vi "Create.vi"(8 "ErrorArray":errorcluster[](array[cluster]), 10 "name or relative path":string="PARTF\\PARTF.ini") -> (0 "ErrorArray":errorcluster[](array[cluster]), 3 "Ref out":refnum<class "Config.lvclass">)   [LabVIEW 2017, in "Framework.lvlib" / "Config.lvclass"]
uses:
  Config.lvclass
  <vilib>/Utility/sysdir.llb/System Directory Type.ctl
  Typedefs/RootDir.ctl
  Typedefs/Logging.ctl
  Typedefs/eLogLvl.ctl
  Config.lvclass/Config.ctl
  Accessors/Write ConfigFilePath.vi
  Accessors/Write Logging.vi
  Accessors/Write PARTF Root Directory.vi
  <vilib>/Utility/config.llb/NI_LVConfig.lvlib
  <userlib>/NIST/NISTErrorLib/NISTErrorLib.lvlib
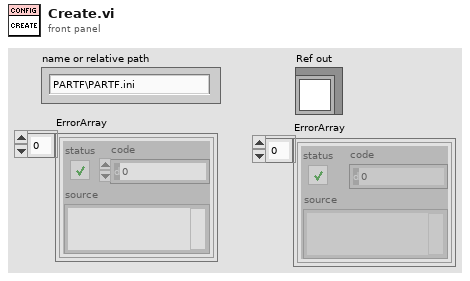
[diagram p1: front panel]
types:
  T1 = typedef "System Directory Type.ctl" = i32
  T2 = typedef "Framework.lvlib/Config.lvclass/eLogLvl.ctl" = enum16{"Normal", "Verbose", "None"}
  T3 = typedef "Framework.lvlib/Config.lvclass/Logging.ctl" = cluster{"eLogLvl":T2, "Log File Path":path, "btnLogFile":bool}
  T4 = typedef "Framework.lvlib/Config.lvclass/RootDir.ctl" = cluster{"pathRootDir":path, "btnOutPath":bool, "OutDir":string, "btnOpenOutputDir":bool, "ScriptDir":string, "btnOpenScriptDir":bool, "TestDir":string, "btnOpenTestDir":bool}
  T5 = cluster{"pathRootDir":path, "OutDir":string, "ScriptDir":string, "TestDir":string}
  T6 = typedef "NI_LVConfig.lvlib/Config Data RefNum.ctl" = refnum<k1>
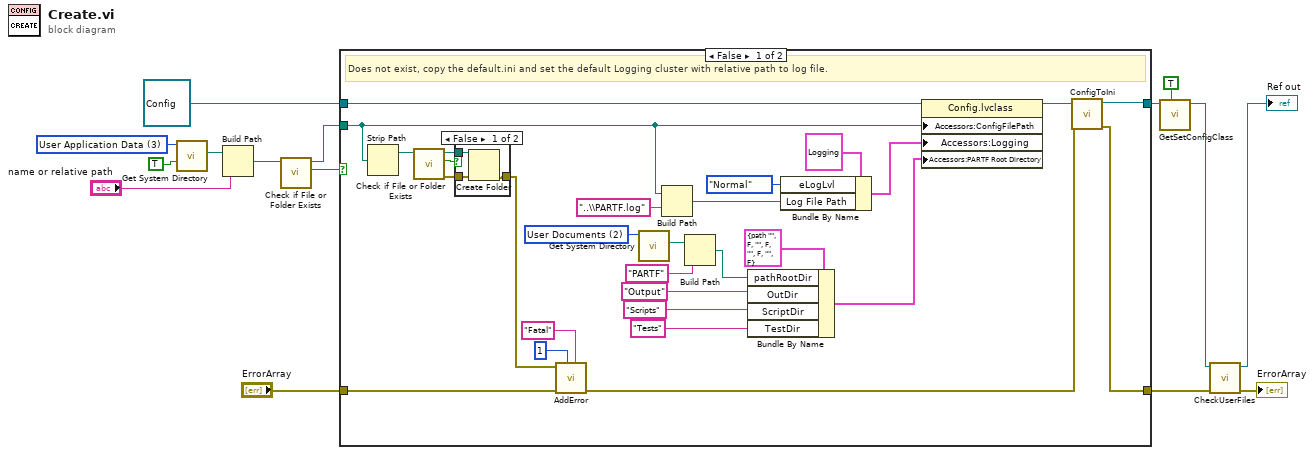
[diagram p0: block diagram]
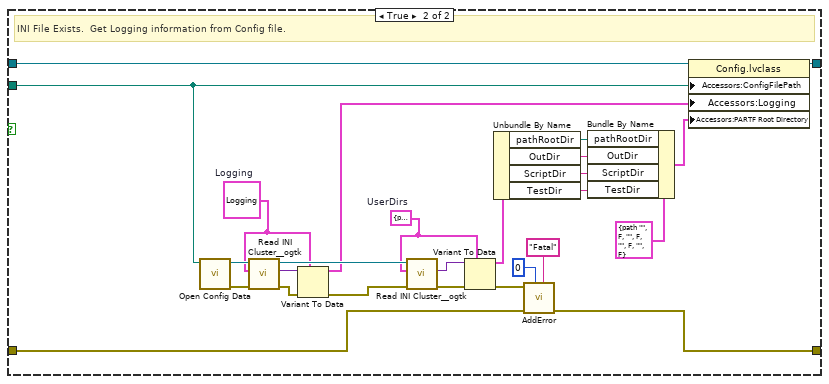
[diagram p3: hidden frame]
diagram:
  w15 = T1 3 items=["User Home"=0, "User Desktop"=1, "User Documents"=2, "User Application Data"=3, "User Preferences"=4, "User Temporary"=5, "Public Documents"=6, "Public Application Data"=7, "Public Preferences"=8, "Public Cache"=13, "System Core Libraries"=9, "System Installed Libraries"=10, "Application Files"=11, "Boot Volume Root"=12] ("system directory type")
  n1 = call <vilib>:"Get System Directory.vi"("create directory if not found? (F)"=TRUE, "system directory type"=w15) -> ("system directory"=w7:path)  [unwired: 9 in]
  n2 = Build Path(base path=w7, name or relative path="name or relative path") -> (appended path=w11:path)
  n3 = call <vilib>:"Check if File or Folder Exists.vi"("path"=w11) -> ("file or folder exists?"=w12:bool, "dup path"=w8:path)  [unwired: 8 in, 1 out]
  n4 = case shown="False" w12 {
    tunnel: w8 -> [w26 w63]
    tunnel: refnum<class "Config.lvclass"> refnum ("Framework.lvlib:Config.lvclass") -> [w43 w73]
    tunnel: [w27 w64] -> w2
    tunnel: "ErrorArray" -> [w24 w60]
    tunnel: [w28 w59] -> w1
    frame False {
      w42 = T1 2 items=["User Home"=0, "User Desktop"=1, "User Documents"=2, "User Application Data"=3, "User Preferences"=4, "User Temporary"=5, "Public Documents"=6, "Public Application Data"=7, "Public Preferences"=8, "Public Cache"=13, "System Core Libraries"=9, "System Installed Libraries"=10, "Application Files"=11, "Boot Volume Root"=12] ("system directory type")
      # "Does not exist, copy the default.ini and set the default Logging cluster with relative path to log file."
      n5 = Strip Path(path=w26) -> (stripped path=w19:path)  [unwired: 1 out]
      n6 = call <vilib>:"Check if File or Folder Exists.vi"("path"=w19) -> ("error out"=w16:errorcluster, "file or folder exists?"=w18:bool, "dup path"=w17:path)  [unwired: 8 in]
      n7 = case shown="False" w18 {
        tunnel: [w46 w47] -> w22
        tunnel: w17 -> [w45 _]
        tunnel: w16 -> [w44 w47]
        frame False {
          n8 = Create Folder(path (use dialog)=w45, error in=w44) -> (error out=w46:errorcluster)  [unwired: 1 in, 2 out]
        }
        frame True {
        }
      }
      n9 = call <userlib>:"AddError.vi"("Severity"="Fatal", "Priority"=u8 1, "ErrorArray"=w24, "error in (no error)"=w22) -> ("ErrorArray"=w23:errorcluster[])  [unwired: 6 in, 1 out]
      n10 = call <vilib>:"Get System Directory.vi"("system directory type"=w42) -> ("system directory"=w41:path)  [unwired: 10 in]
      n11 = Build Path(base path=w26, name or relative path="..\\PARTF.log") -> (appended path=w32:path)
      n12 = Build Path(base path=w41, name or relative path="PARTF") -> (appended path=w38:path)
      n13 = Bundle By Name(cluster=T4 {"pathRootDir"=path "", "btnOutPath"=FALSE, "OutDir"="", "btnOpenOutputDir"=FALSE, "ScriptDir"="", "btnOpenScriptDir"=FALSE, "TestDir"="", "btnOpenTestDir"=FALSE} ("PARTF Root Directory"), "pathRootDir"=w38, "OutDir"="Output", "ScriptDir"="Scripts", "TestDir"="Tests" ("ScriptDir")) -> (w35:T4)
      n14 = Bundle By Name(cluster=T3 {"eLogLvl"=enum."Normal", "Log File Path"=path "C:/Users/gra1/AppData/Local/Framework/Framework.log", "btnLogFile"=FALSE} ("Logging"), "eLogLvl"=eLogLvl."Normal", "Log File Path"=w32) -> (w30:T3)
      n15 = property class="Config.lvclass"(reference=w43, "Accessors:ConfigFilePath"=w26, "Accessors:Logging"=w30, "Accessors:PARTF Root Directory"=w35) -> (reference out=w29:refnum<class "Config.lvclass">)  [unwired: 1 in, 1 out]
      n16 = call "ConfigToIni.vi"("Error In"=w23, "ConfigRef"=w29) -> ("Error Out"=w28:errorcluster[], "ConfigRef"=w27:refnum<class "Config.lvclass">)  [unwired: 8 in]
    }
    frame True {
      w56 = T3 {"eLogLvl"=enum."Normal", "Log File Path"=path "C:/Users/gra1/AppData/Local/Framework/Framework.log", "btnLogFile"=FALSE}  # Logging
      w57 = T5 {"pathRootDir"=path "", "OutDir"="", "ScriptDir"="", "TestDir"=""}  # UserDirs
      # "INI File Exists.  Get Logging information from Config file."
      n17 = call <vilib>:"Open Config Data.vi"("configuration file path"=w63) -> ("error out"=w72:errorcluster, "refnum"=w71:T6)  [unwired: 8 in, 1 out]
      n18 = call <userlib>:"Read INI Cluster__ogtk.vi"("error in (no error)"=w72, "INI Fomatted Cluster Type"=w56, "refnum"=w71) -> ("error out"=w70:errorcluster, "INI Fomatted Cluster"=w69:variant, "dup refnum"=w68:T6)  [unwired: 4 in, 2 out]
      n19 = Variant To Data(error in=w70, type=w56, Variant=w69) -> (data=w55:T3, error out=w67:errorcluster)
      n20 = call <userlib>:"Read INI Cluster__ogtk.vi"("error in (no error)"=w67, "INI Fomatted Cluster Type"=w57, "refnum"=w68) -> ("error out"=w66:errorcluster, "INI Fomatted Cluster"=w65:variant)  [unwired: 4 in, 3 out]
      n21 = Variant To Data(error in=w66, type=w57, Variant=w65) -> (data=w54:T5, error out=w58:errorcluster)
      n22 = Unbundle By Name(w54) -> ("pathRootDir"=w52:path, "OutDir"=w51:string, "ScriptDir"=w50:string, "TestDir"=w49:string)
      n23 = call <userlib>:"AddError.vi"("Severity"="Fatal", "Priority"=u8 0, "ErrorArray"=w60, "error in (no error)"=w58) -> ("ErrorArray"=w59:errorcluster[])  [unwired: 6 in, 1 out]
      n24 = Bundle By Name(cluster=T4 {"pathRootDir"=path "", "btnOutPath"=FALSE, "OutDir"="", "btnOpenOutputDir"=FALSE, "ScriptDir"="", "btnOpenScriptDir"=FALSE, "TestDir"="", "btnOpenTestDir"=FALSE} ("PARTF Root Directory"), "pathRootDir"=w52, "OutDir"=w51, "ScriptDir"=w50, "TestDir"=w49) -> (w48:T4)
      n25 = property class="Config.lvclass"(reference=w73, "Accessors:ConfigFilePath"=w63, "Accessors:Logging"=w55, "Accessors:PARTF Root Directory"=w48) -> (reference out=w64:refnum<class "Config.lvclass">)  [unwired: 1 in, 1 out]
    }
  }
  n26 = call "GetSetConfigClass.vi"("Set (f)"=TRUE, "Ref in"=w2) -> ("Ref out"=w5:refnum<class "Config.lvclass">)  [unwired: 9 in]
  n27 = call "CheckUserFiles.vi"("ErrorArray"=w1, "Config in"=w5) -> ("ErrorArray"=→"ErrorArray":errorcluster[], "Config out"=→"Ref out":refnum<class "Config.lvclass">)  [unwired: 8 in]
